vi "Pot Line of Points.vi"(6 "Potting Parameters":T1={"Curing Param A"=0.0, "Curing Param B"=0.0, "Speed Nominal"=-1.0, "Time Nominal"=0.0, "Turn-on Time"=0.0, "Turn-off Time"=0.0, "Safe Height Offset"=0.0, "Tip Height"=0.0, "Pot Length Scale"=0.0, "Number of dots"=1.0, "Distance between dots"=0.0}, 7 "Potting Surface Type":T2, 8 "error in (no error)":errorcluster, 9 "End Position":refnum<class "Vec3d Class.lvclass">, 10 "Start Position":refnum<class "Vec3d Class.lvclass">, 11 "SyringeTool Class in":refnum<class "SyringeTool Class.lvclass">) -> (0 "error out":errorcluster, 3 "SyringeTool Class out":refnum<class "SyringeTool Class.lvclass">)   [LabVIEW 2017, in "SyringeTool Class.lvclass"]
uses:
  SyringeTool Class.lvclass
  Config Manager Class/Type Definitions/Potting Surface Type.ctl
  Config Manager Class/Type Definitions/Potting Parameters.ctl
  Vec3d Class/Vec3d Class.lvclass
  Utils/Type Definitions/3d Point.ctl
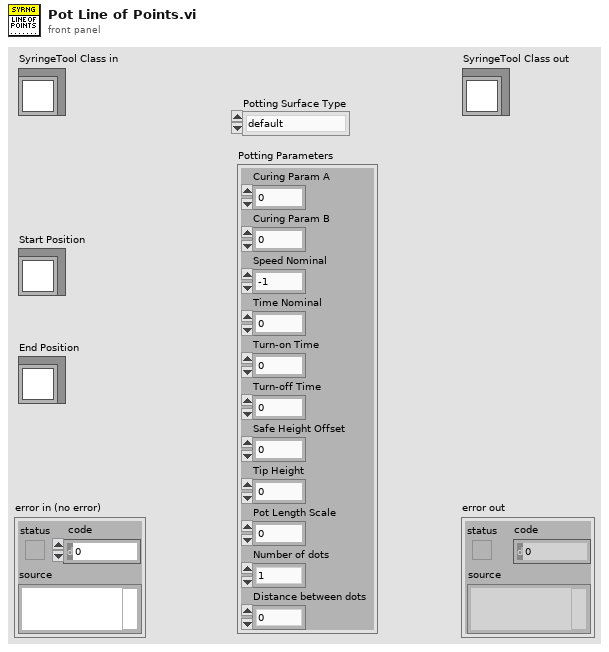
[diagram p1: front panel]
types:
  T1 = typedef "Potting Parameters.ctl" = cluster{"Curing Param A":dbl, "Curing Param B":dbl, "Speed Nominal":dbl, "Time Nominal":dbl, "Turn-on Time":dbl, "Turn-off Time":dbl, "Safe Height Offset":dbl, "Tip Height":dbl, "Pot Length Scale":dbl, "Number of dots":dbl, "Distance between dots":dbl}
  T2 = typedef "Potting Surface Type.ctl" = enum16{"default", "hdi_edge_pads", "bbm_edge_pads", "address_pads"}
  T3 = typedef "3d Point.ctl" = cluster{"Point":refnum<class "Vec3d Class.lvclass">, "Enable":bool}
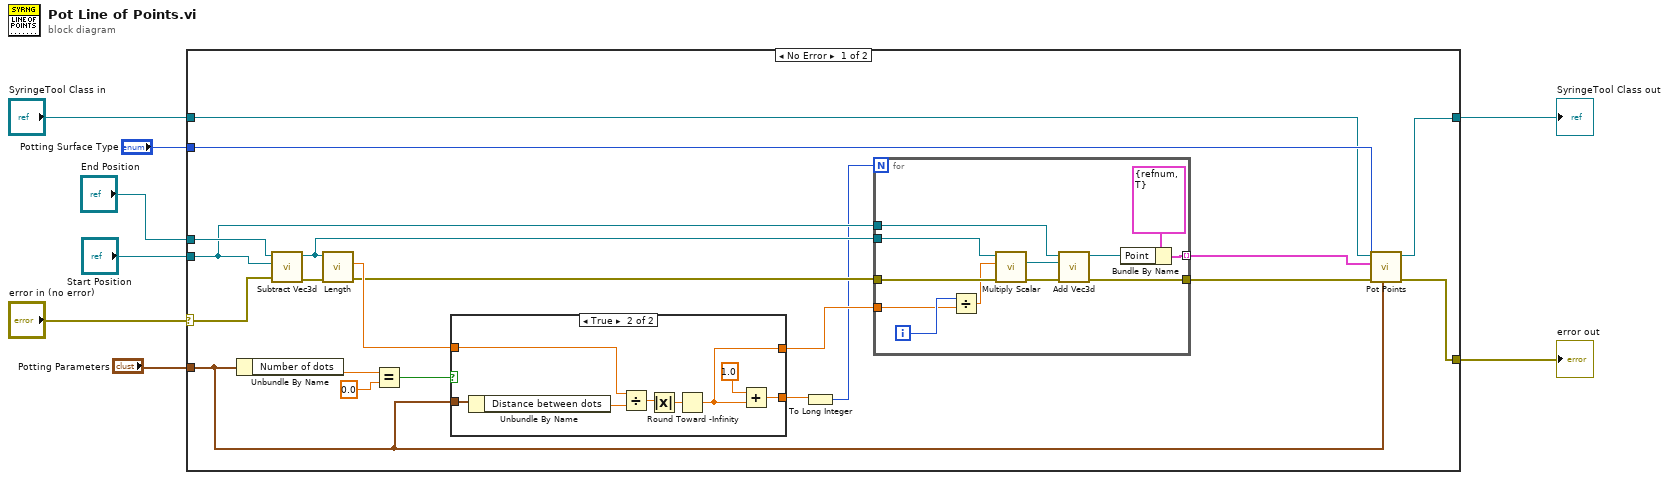
[diagram p0: block diagram]
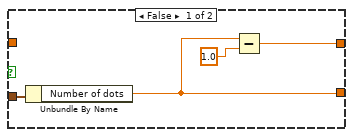
[diagram p2: hidden frame]
diagram:
  n1 = case shown="No Error" "error in (no error)" {
    selector: "error in (no error)" -> [w21 w54]
    tunnel: [w18 w53] -> w6
    tunnel: "SyringeTool Class in" -> [w19 w53]
    tunnel: "Start Position" -> [w16 _]
    tunnel: "End Position" -> [w17 _]
    tunnel: "Potting Surface Type" -> [w22 _]
    tunnel: [w20 w54] -> w4
    tunnel: "Potting Parameters" -> [w12 _]
    frame No Error {
      n2 = Unbundle By Name(w12) -> ("Number of dots"=w15:dbl)
      n3 = call "Subtract Vec3d.vi"("error in (no error)"=w21, "Vec3d in 2"=w16, "Vec3d in 1"=w17) -> ("error out"=w28:errorcluster, "Vec3d Class out"=w26:refnum<class "Vec3d Class.lvclass">)  [unwired: 7 in]
      n4 = call-dynamic "Length.vi"("error in"=w28, "Vec3d in"=w26) -> ("error out"=w24:errorcluster, "Length"=w25:dbl)  [unwired: 7 in, 1 out]
      n5 = Equal?(x=w15, y=0.0) -> (x = y?=w13:bool)
      n6 = case shown="True" w13 {
        tunnel: w25 -> [_ w34]
        tunnel: w12 -> [w32 w38]
        tunnel: [w31 w35] -> w9
        tunnel: [w30 w33] -> w11
        frame False {
          n7 = Unbundle By Name(w32) -> ("Number of dots"=w31:dbl)
          n8 = Subtract(x=w31, y=1.0) -> (x-y=w30:dbl)
        }
        frame True {
          n9 = Unbundle By Name(w38) -> ("Distance between dots"=w37:dbl)
          n10 = Divide(x=w34, y=w37) -> (x/y=w39:dbl)
          n11 = Absolute Value(x=w39) -> (abs(x)=w40:dbl)
          n12 = Round Toward -Infinity(1:w40) -> (0:w33:dbl)
          n13 = Add(x=1.0, y=w33) -> (x+y=w35:dbl)
        }
      }
      n14 = To Long Integer(number=w9) -> (32bit integer=w10:i32)
      n15 = for {
        N: w10 -> [_]
        tunnel: [w52] -> w27 mode=indexing
        tunnel: w26 -> [w50]
        tunnel: w24 -> [w49]
        tunnel: [w47] -> w23
        tunnel: w16 -> [w45]
        tunnel: w11 -> [w41]
        i -> [w42]
        n16 = Divide(x=w42, y=w41) -> (x/y=w43:dbl)
        n17 = call-dynamic "Multiply Scalar.vi"("error in"=w49, "Scale"=w43, "Vec3d in"=w50) -> ("error out"=w48:errorcluster, "Vec3d out"=w44:refnum<class "Vec3d Class.lvclass">)  [unwired: 7 in]
        n18 = call-dynamic "Add Vec3d.vi"("error in (no error)"=w48, 10:"Vec3d Class in"=w44, 11:"Vec3d Class in"=w45) -> ("error out"=w47:errorcluster, "Vec3d Class out"=w46:refnum<class "Vec3d Class.lvclass">)  [unwired: 7 in]
        n19 = Bundle By Name(cluster=T3 {"Point"=refnum, "Enable"=TRUE} ("3d Point"), "Point"=w46) -> (w52:T3)
      }
      n20 = call-dynamic "Pot Points.vi"("Potting Parameters"=w12, "Potting Surface Type"=w22, "error in"=w23, "Points"=w27, "SyringeTool in"=w19) -> ("error out"=w20:errorcluster, "SyringeTool out"=w18:refnum<class "SyringeTool Class.lvclass">)  [unwired: 5 in]
    }
    frame Error {
    }
  }
  "error out" <- w4
  "SyringeTool Class out" <- w6
